vi "Set Tester Rx.vi"(8 "error in (no error)":errorcluster, 11 "Station Actor in":refnum<class "Station Actor.lvclass">) -> (0 "error out":errorcluster, 3 "Station Actor out":refnum<class "Station Actor.lvclass">)   [LabVIEW 2019, in "Station Actor.lvlib" / "Station Actor.lvclass"]
uses:
  Station Actor.lvclass
  Station Actor.lvclass/Station Actor.ctl
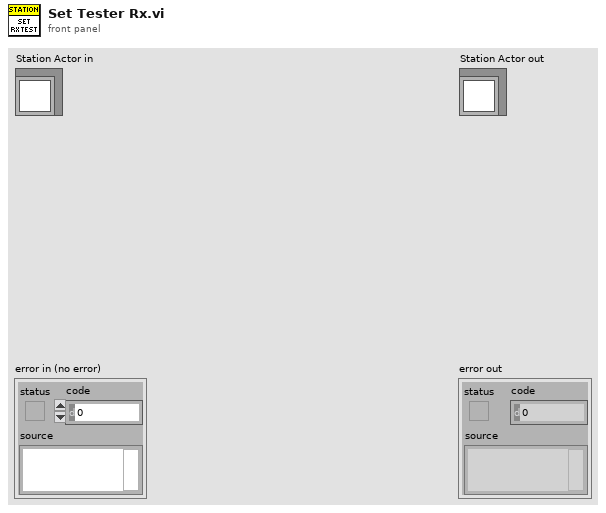
[diagram p1: front panel]
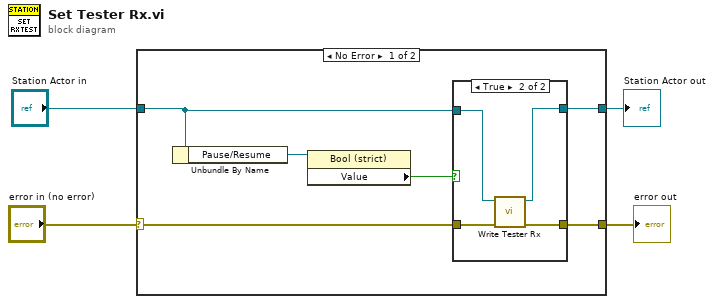
[diagram p0: block diagram]
diagram:
  n1 = case shown="No Error" "error in (no error)" {
    selector: "error in (no error)" -> [w8 w18]
    tunnel: [w7 w18] -> w3
    tunnel: [w5 w17] -> w1
    tunnel: "Station Actor in" -> [w6 w17]
    frame No Error {
      n2 = Unbundle By Name(w6) -> ("Pause/Resume"=w10:refnum<vi>)
      n3 = property class="Bool (strict)"(reference=w10) -> ("Value"=w9:bool)  [unwired: 1 in, 2 out]
      n4 = case shown="True" w9 {
        tunnel: w8 -> [w12 w16]
        tunnel: [w12 w15] -> w7
        tunnel: w6 -> [w11 w14]
        tunnel: [w11 w13] -> w5
        frame False {
        }
        frame True {
          n5 = call "Write Tester Rx.vi"("error in (no error)"=w16, "Panel in"=w14) -> ("error out"=w15:errorcluster, "Panel out"=w13:refnum<class "Station Actor.lvclass">)  [unwired: 8 in]
        }
      }
    }
    frame Error {
    }
  }
  "error out" <- w3
  "Station Actor out" <- w1
